vi "qDFH.vi"(0 "System no.":i32=1 min=1 max=4 step=1, 2 "Axes to query":string[](array[string]), 3 "All axes?":bool, 4 "Axis identifier?":bool=TRUE, 5 "error in":errorcluster) -> (14 "Home position":dbl[](array[numeric]) format="%.6f", 19 "error out":errorcluster)   [LabVIEW 2026]
doc: "Returns the difference between the current home position and the absolute or initial zero point (default home position) for each of the queried axes.\n\nC-702, C-848, C-877, C-880, C-884, E-517, E-518, E-871, E-873, E-874, Hydra, Pollux, Mercury, Mercury_GCS: If All axes? = TRUE, then Axis identifier? can be FALSE \n\nC-843, C-843.PM, C-844, C-865, C-866, E-710, E-761: If All axes? = TRUE, then Axis identifier? must be TRUE\n\nC-867, Mercury_GCS: If All axes? = TRUE, then Axis identifier? can be FALSE. \n\nC-880K005: VI only supported when called through PI_Multix.vi\n\nE-755: If All axes? = TRUE, then Axis identifier? can be FALSE. Command not available for E-755.101."
panel:
  # "Returns the difference between the current home position and \nthe absolute or initial zero point (default home position) for each \nof the queried axes."
  # "If all axes: use"
  # "Query"
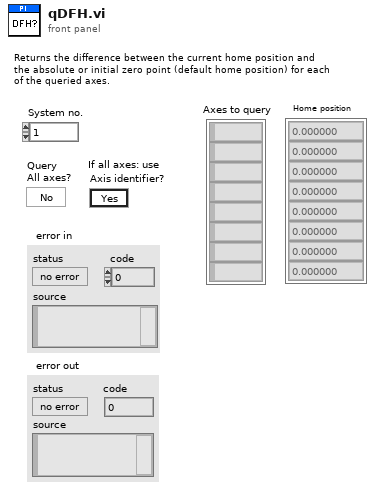
[diagram p1: front panel]
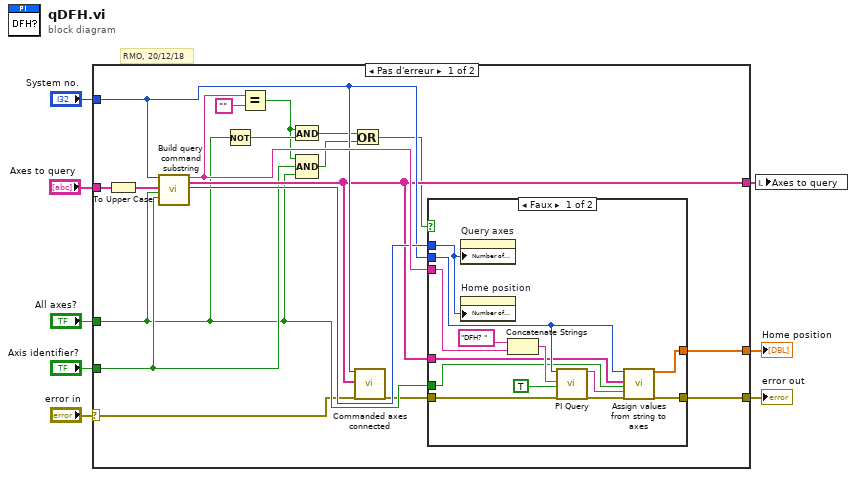
[diagram p0: block diagram]
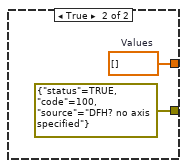
[diagram p2: hidden frame]
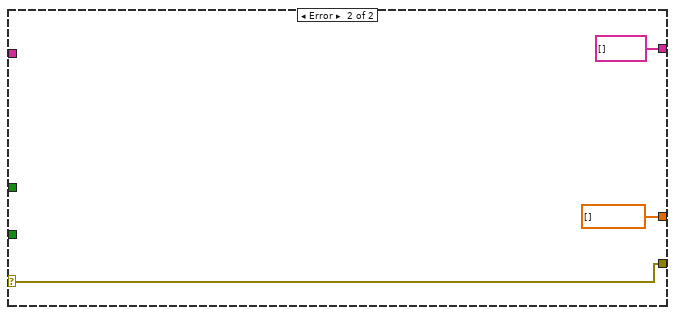
[diagram p3: hidden frame]
diagram:
  # "RMO, 20/12/18"
  n1 = case shown="Pas d'erreur" "error in" {
    selector: "error in" -> [w11 w42]
    tunnel: [w26 dbl[] [] ("Values")] -> w8
    tunnel: "Axes to query" -> [w25 _]
    tunnel: [w12 w42] -> w6
    tunnel: "System no." -> [w20 _]
    tunnel: [w19 string[] [] ("Axes to query out")] -> w4
    tunnel: "Axis identifier?" -> [w15 _]
    tunnel: "All axes?" -> [w14 _]
    frame No Error {
      n2 = To Upper Case(1:w25) -> (0:w23:string[])
      n3 = call "Build query command substring.vi"("System no."=w20, "Axes to query in"=w23, "Query\nAll axes?"=w14, "For all axes: use\nAxis identifier?"=w15) -> ("Command substring"=w22:string, "Axes to query out"=w19:string[], "Number of rows"=w21:u32)  [unwired: 2 in, 11 out]
      n4 = Not(x=w14) -> (.not. x?=w18:bool)
      n5 = Equal?(x=w22, y="" ("x")) -> (x = y?=w16:bool)
      n6 = And(x=w16, y=w18) -> (x .and. y?=w17:bool)
      n7 = Compound Arithmetic op=AND(w16, w15, w14) -> (w13:bool)
      n8 = Or(x=w17, y=w13) -> (x .or. y?=w9:bool)
      n9 = call "Commanded axes connected.vi"("System no."=w20, "Commanded axes"=w19, "error in"=w11) -> ("error out"=w10:errorcluster)  [unwired: 1 in, 15 out]
      n10 = case shown="Faux" w9 {
        tunnel: [w36 w40] -> w26
        tunnel: w22 -> [w35 _]
        tunnel: w21 -> [w34 _]
        tunnel: w20 -> [w33 _]
        tunnel: w19 -> [w32 _]
        tunnel: w14 -> [w31 _]
        tunnel: [w30 errorcluster {"status"=TRUE, "code"=100, "source"="DFH? no axis specified"} ("error out")] -> w12
        tunnel: w10 -> [w29 _]
        frame False {
          n11 = property on="Query axes" class="Tabl (strict)"("Number of Rows"=w34) -> ()  [unwired: 2 in, 2 out]
          n12 = property on="Home position" class="Tabl (strict)"("Number of Rows"=w34) -> ()  [unwired: 2 in, 2 out]
          n13 = Concatenate Strings("DFH? ", w35) -> (w37:string)
          n14 = call "PI Query.vi"("System no."=w33, "String to send"=w37, "Attach termination char.?"=TRUE ("Attach Linefeed?"), "error in"=w29) -> ("String read"=w27:string, "error out"=w28:errorcluster)  [unwired: 3 in, 11 out]
          n15 = call "Assign values from string to axes.vi"("System no."=w33, "Queried axes"=w32, "All axes queried?"=w31, "Input String"=w27, "error in"=w28) -> ("Values"=w36:dbl[], "error out"=w30:errorcluster)  [unwired: 4 in, 9 out]
        }
        frame True {
          w40 = dbl[] []  # Values
        }
      }
    }
    frame Error {
    }
  }
  "error out" <- w6
  "Home position" <- w8
  n16 = local write "Axes to query"(w4) -> ()
